vi "Write.vi"(8 "error in (no error)":errorcluster, 10 "Array":string[][](array[string]), 11 "Save as csv in":refnum<class "Save as csv.lvclass">) -> (0 "error out":errorcluster, 3 "Save as csv out":refnum<class "Save as csv.lvclass">)   [LabVIEW 2020, in "Save as csv.lvclass"]
uses:
  Save as csv.lvclass
  Saving OO.lvclass
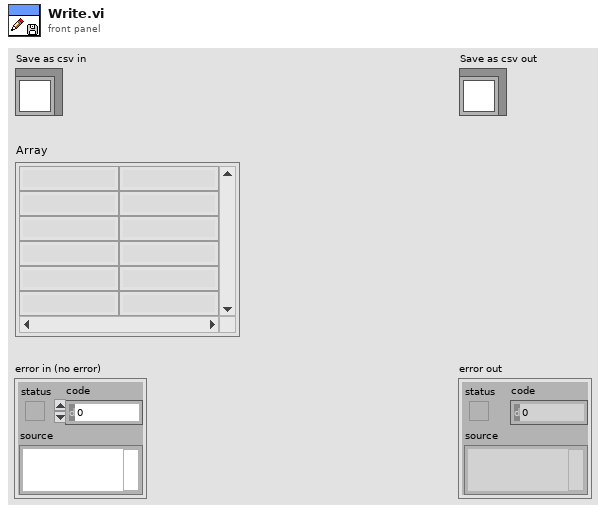
[diagram p1: front panel]
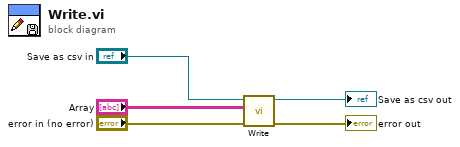
[diagram p0: block diagram]
diagram:
  n1 = call-parent "Write.vi"("error in (no error)"="error in (no error)", "Array"="Array", "Saving OO in"="Save as csv in") -> ("error out"=→"error out":errorcluster, "Saving OO out"=→"Save as csv out":refnum<class "Save as csv.lvclass">)  [unwired: 7 in]
